vi "McPherson Emergency Stop.vi"(6 "VISA Resource Name":refnum<visa-resource-name>) -> (0 "error out":errorcluster, 2 "dup VISA Resource Name":refnum<visa-resource-name>)   [LabVIEW 2021]
uses:
  Serial Instruments/Serial Support VISA.llb/Serial Actions.ctl
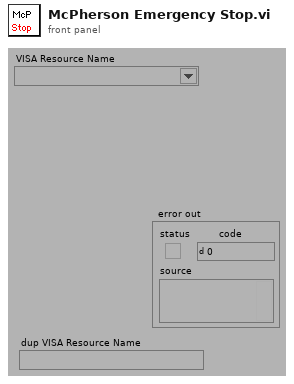
[diagram p1: front panel]
types:
  T1 = typedef "Serial Actions.ctl" = enum16{"Init", "Break", "Clear Buffer", "Write", "Read", "N Bytes", "Lock", "Unlock", "Close"}
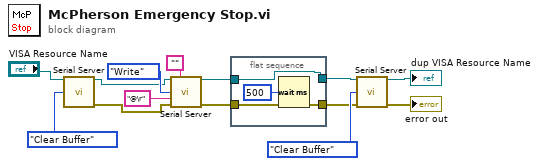
[diagram p0: block diagram]
diagram:
  n1 = call "Serial Server.vi"("VISA Resource Name"="VISA Resource Name", "Action"=Serial_Actions."Clear Buffer") -> ("dup VISA Resource Name"=w6:refnum<visa-resource-name>, "error out"=w7:errorcluster)  [unwired: 9 in, 3 out]
  n2 = call "Serial Server.vi"("VISA Resource Name"=w6, "EOT Chars (cr/lf)"="", "Action"=Serial_Actions."Write", "String To Send"="@\r", "error in (no error)"=w7) -> ("dup VISA Resource Name"=w2:refnum<visa-resource-name>, "error out"=w4:errorcluster)  [unwired: 6 in, 3 out]
  n3 = flat-sequence {
    tunnel: w4 -> [w16]
    tunnel: [w16] -> w3
    tunnel: [w15] -> w1
    tunnel: w2 -> [w15]
    frame #0 {
      n4 = Wait (ms)(milliseconds to wait=u32 500) -> ()  [unwired: 1 out]
    }
  }
  n5 = call "Serial Server.vi"("VISA Resource Name"=w1, "Action"=Serial_Actions."Clear Buffer", "error in (no error)"=w3) -> ("dup VISA Resource Name"=→"dup VISA Resource Name":refnum<visa-resource-name>, "error out"=→"error out":errorcluster)  [unwired: 8 in, 3 out]
